vi "JKI.Robot.SMO.SetJointRotation.Private.vi"(8 "error in (no error)":errorcluster, 9 "Robot Position.Claw Value":dbl format="%#_13g", 10 "Joint":T1, 11 "JKI.Robot.SMO":refnum<class "JKI.Robot.SMO.lvclass">) -> (0 "error out":errorcluster, 3 "JKI.Robot.SMO out":refnum<class "JKI.Robot.SMO.lvclass">)   [LabVIEW 2015, in "JKI.Robot.SMO.lvclass"]
doc: "---------------------------------------------------------------\nJKI State Machine Objects™\nhttp://jki.net/state-machine-objects/\nCopyright (C) 2005-2015, JKI <info@jki.net>\nALL RIGHTS RESERVEDJKI State Machine Objects (SMO) 1.0.0.5\nJKI - JKI\nCopyright (c) 2016, JKI"
uses:
  JKI.Robot.SMO.lvclass
  Typedefs/JointType--Enum.ctl
  JKI.Robot.SMO.lvclass/JKI.Robot.SMO.ctl
  Typedefs/DataChanged--EventData--Cluster.ctl
  Typedefs/RobotPosition--Cluster.ctl
panel:
  # "For instructions on how to use the JKI State Machine Objects, examples and video tutorials, visit:\nhttp://jki.net/state-machine-objects/\n\nJKI State Machine Objects™\nhttp://jki.net/state-machine-objects/\nCopyright (C) 2005-2015, JKI <info@jki.net>\nALL RIGHTS RESERVED"
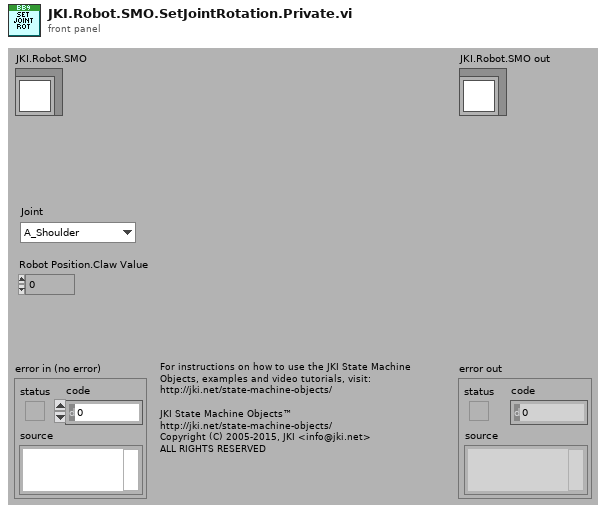
[diagram p1: front panel]
types:
  T1 = typedef "JointType--Enum.ctl" = enum16{"A_Shoulder", "B_Elbow", "C_Wrist", "D_Base"}
  T2 = typedef "JKI.Robot.SMO.lvclass/DataChanged--EventData--Cluster.ctl" = cluster{"Timestamp":timestamp, "Old Position":T3, "New Position":T3}
  T3 = typedef "RobotPosition--Cluster.ctl" = cluster{"Claw":dbl, "JointA":dbl, "JointB":dbl, "JointC":dbl, "JointD":dbl}
  T4 = typedef "JKI.Robot.SMO.lvclass/PrivateData--Ref.ctl" = refnum<data-value>
  T5 = typedef "JKI.Robot.SMO.lvclass/PrivateData--Cluster.ctl" = cluster{"Configuration":T6, "Public Events":T7, "Robot Position":T3, "Private Events":T8}
  T6 = typedef "JKI.Robot.SMO.lvclass/Configuration--Cluster.ctl" = cluster{"Suffix":string}
  T7 = typedef "JKI.Robot.SMO.lvclass/PublicEvents--Cluster.ctl" = cluster{"Data Changed":refnum<user-event>}
  T8 = typedef "JKI.Robot.SMO.lvclass/PrivateEvents--Cluster.ctl" = cluster{"SetGrabberPosition":refnum<user-event>, "SetJointRotation":refnum<user-event>}
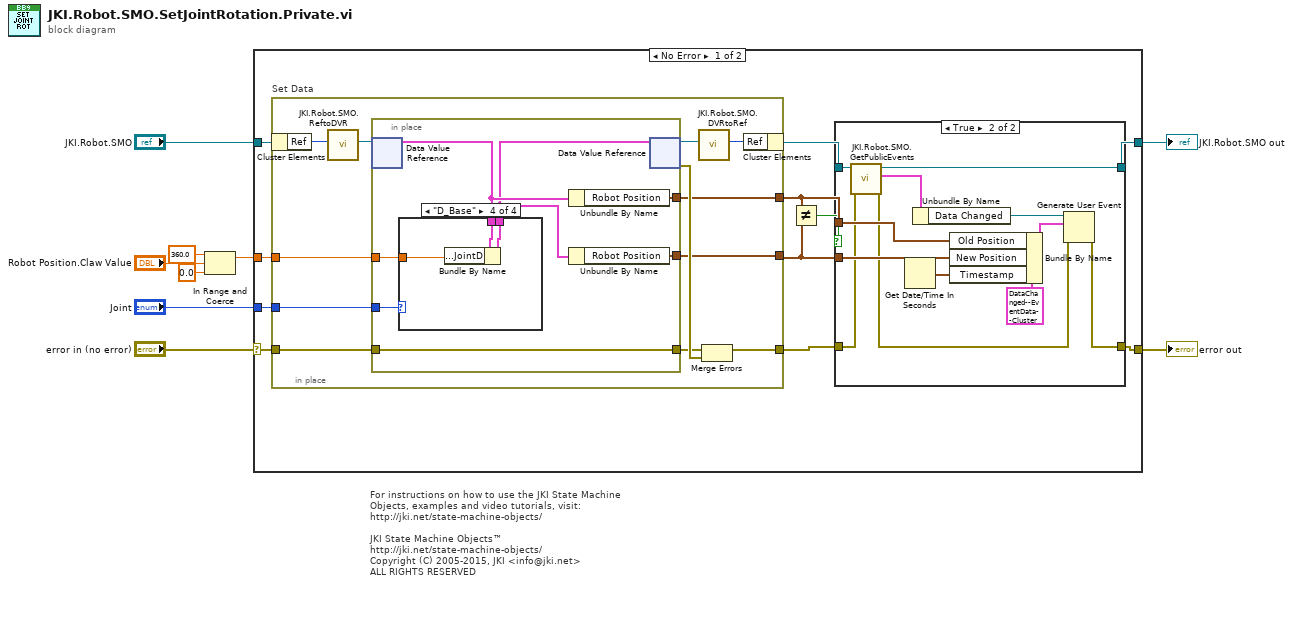
[diagram p0: block diagram]
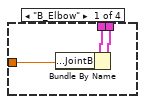
[diagram p3: hidden frame]
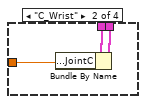
[diagram p4: hidden frame]
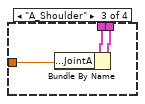
[diagram p5: hidden frame]
diagram:
  # "For instructions on how to use the JKI State Machine Objects, examples and video tutorials, visit:\nhttp://jki.net/state-machine-objects/\n\nJKI State Machine Objects™\nhttp://jki.net/state-machine-objects/\nCopyright (C) 2005-2015, JKI <info@jki.net>\nALL RIGHTS RESERVED"
  n1 = In Range and Coerce(upper limit=360.0, x="Robot Position.Claw Value", lower limit=0.0) -> (coerced(x)=w3:dbl)  [unwired: 1 out]
  n2 = case shown="No Error" "error in (no error)" {
    selector: "error in (no error)" -> [w19 w66]
    tunnel: "JKI.Robot.SMO" -> [w20 w67]
    tunnel: [w17 w66] -> w8
    tunnel: [w12 w67] -> w7
    tunnel: w3 -> [w11 _]
    tunnel: "Joint" -> [w10 _]
    frame No Error {
      n3 = in-place "Set Data" {
        in-place-border: w19 -> [w46]
        in-place-border: [w43] -> w18
        in-place-border: [w42] -> w14
        in-place-border: [w41] -> w15
        in-place-border: w11 -> [w36]
        in-place-border: w10 -> [w35]
        n4 = in-place-cluster #1(w20) -> ("Ref"=w40:u32)
        n5 = call "JKI.Robot.SMO.ReftoDVR.vi"("Ref"=w40) -> ("Ref"=w39:T4)  [unwired: 10 in]
        n6 = in-place {
          in-place-border: w46 -> [w53]
          in-place-border: [w53] -> w44
          in-place-border: [w49] -> w42
          in-place-border: [w52] -> w41
          in-place-border: w36 -> [w48]
          in-place-border: w35 -> [w47]
          n7 = in-place-dvr #2(w39) -> (w51:T5)  [unwired: 1 out]
          n8 = case shown="\"D_Base\"" w47 {
            tunnel: w51 -> [w56 w59 w62 w65]
            tunnel: [w55 w58 w61 w64] -> w50
            tunnel: w48 -> [w54 w57 w60 w63]
            frame "B_Elbow" {
              n9 = Bundle By Name(cluster=w56, "Robot Position.JointB"=w54) -> (w55:T5)
            }
            frame "C_Wrist" {
              n10 = Bundle By Name(cluster=w59, "Robot Position.JointC"=w57) -> (w58:T5)
            }
            frame "A_Shoulder" {
              n11 = Bundle By Name(cluster=w62, "Robot Position.JointA"=w60) -> (w61:T5)
            }
            frame "D_Base" {
              n12 = Bundle By Name(cluster=w65, "Robot Position.JointD"=w63) -> (w64:T5)
            }
          }
          n13 = Unbundle By Name(w51) -> ("Robot Position"=w52:T3)
          n14 = Unbundle By Name(w50) -> ("Robot Position"=w49:T3)
          n15 = in-place-dvr #2(w50) -> (w38:T4, w45:errorcluster)
        }
        n16 = call "JKI.Robot.SMO.DVRtoRef.vi"("Ref"=w38) -> ("Ref"=w37:u32)  [unwired: 10 in]
        n17 = Merge Errors(w44, w45) -> (w43:errorcluster)
        n18 = in-place-cluster #1("Ref"=w37) -> (w16:refnum<class "JKI.Robot.SMO.lvclass">)
      }
      n19 = Not Equal?(x=w15, y=w14) -> (x != y?=w13:bool)
      n20 = case shown="True" w13 {
        tunnel: w18 -> [w21 w26]
        tunnel: w15 -> [_ w31]
        tunnel: w14 -> [_ w30]
        tunnel: [w21 w28] -> w17
        tunnel: w16 -> [w22 w27]
        tunnel: [w22 w24] -> w12
        frame False {
        }
        frame True {
          n21 = call "JKI.Robot.SMO.GetPublicEvents.vi"("error in (no error)"=w26, "JKI.Robot.SMO"=w27) -> ("error out"=w25:errorcluster, "SMO.ByRefWithEvents Public Events"=w23:T7, "JKI.Robot.SMO out"=w24:refnum<class "JKI.Robot.SMO.lvclass">)  [unwired: 7 in]
          n22 = Get Date/Time In Seconds() -> (seconds since 1Jan1904=w29:timestamp)
          n23 = Unbundle By Name(w23) -> ("Data Changed"=w34:refnum<user-event>)
          n24 = Bundle By Name(cluster=T2 {"Timestamp"=timestamp(0 s since 1904-01-01), "Old Position"={"Claw"=0.5192802056555269, "JointA"=347.1752980785341, "JointB"=280.93136534375475, "JointC"=30.749358432304007, "JointD"=30.749358432304007}, "New Position"={"Claw"=0.5192802056555269, "JointA"=347.1752980785341, "JointB"=280.93136534375475, "JointC"=30.749358432304007, "JointD"=30.749358432304007}} ("event data"), "Old Position"=w31, "New Position"=w30, "Timestamp"=w29) -> (w32:T2)
          n25 = Generate User Event(user event=w34, event data cluster=w32, error in=w25) -> (error out=w28:errorcluster)  [unwired: 1 in, 1 out]
        }
      }
    }
    frame Error {
    }
  }
  "error out" <- w8
  "JKI.Robot.SMO out" <- w7
